vi "oax_Path Error Handle.vi"(0 "File Path (.dat)":path, 1 "Ring":u16(ring) items=["Load .wav file", "Load .dat file", "Load tachless file", "Load .ssp file"], 5 "Tacho File Path (.wav)":path, 7 "Vibration File Path (.wav)":path, 9 "Simulated File Path (.ssp)":path, 11 "error In":errorcluster) -> (4 "Error":bool, 15 "error Out":errorcluster)   [LabVIEW 2017]
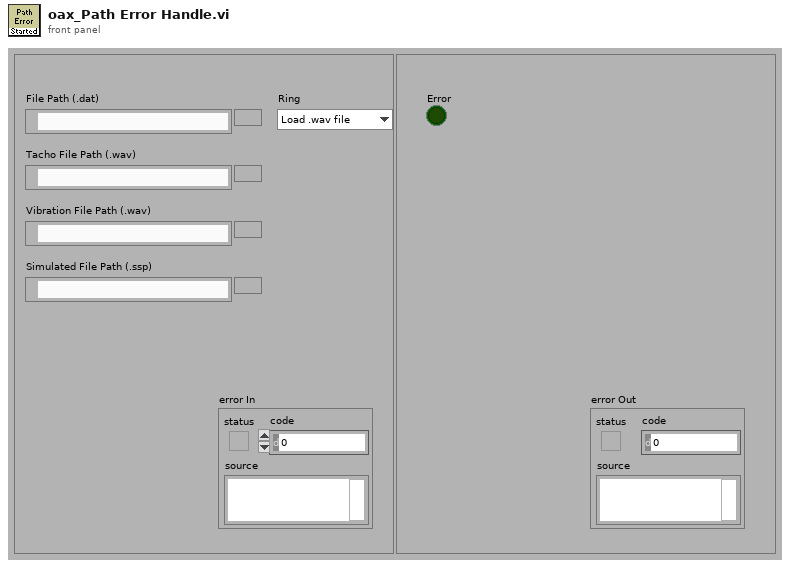
[diagram p1: front panel]
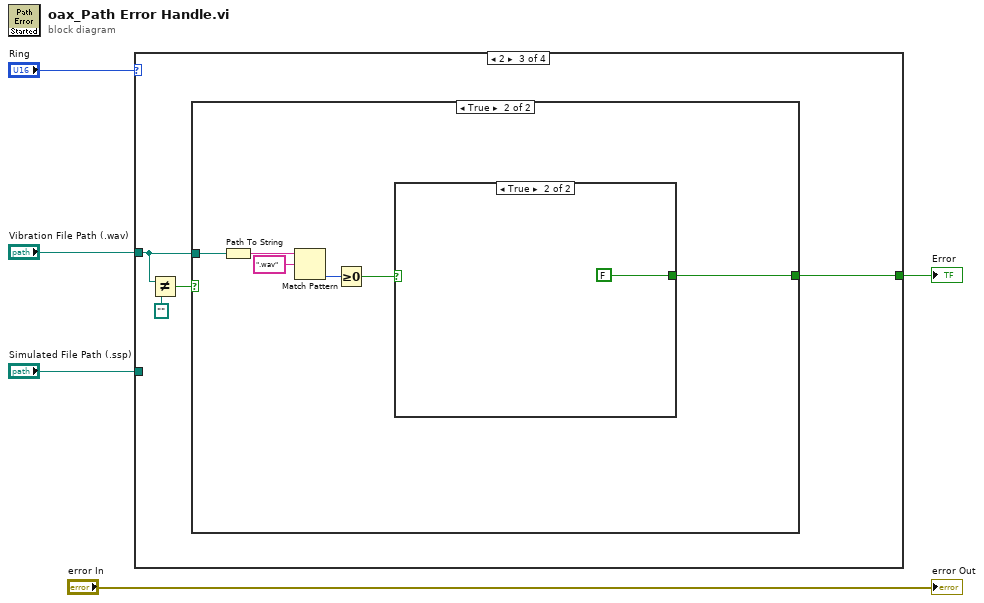
[diagram p0: block diagram]
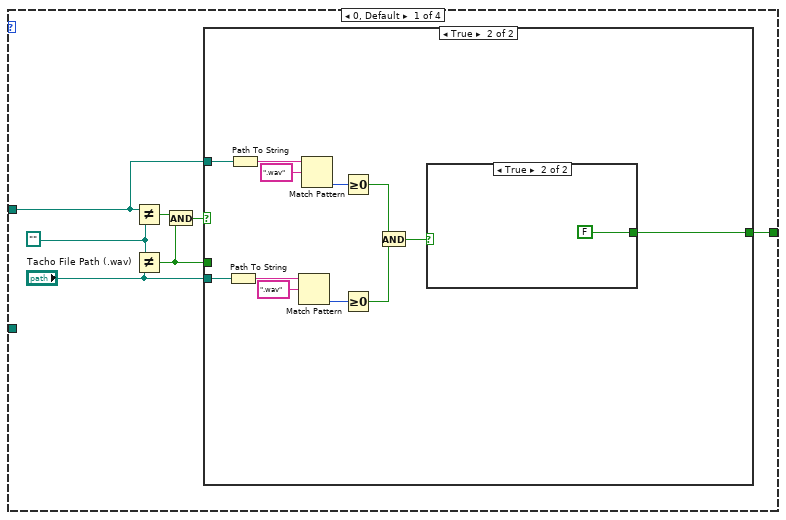
[diagram p2: hidden frame]
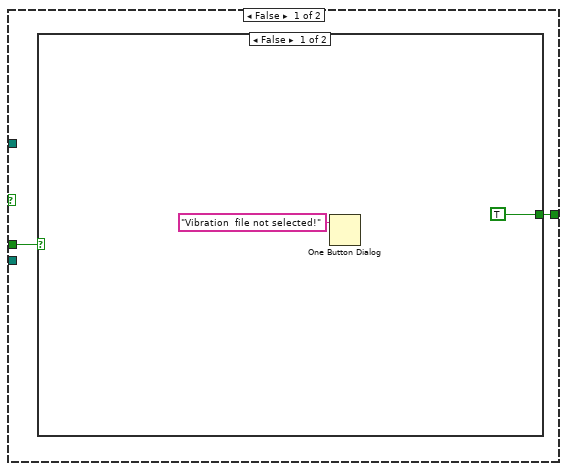
[diagram p3: hidden frame]
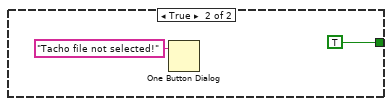
[diagram p4: hidden frame]
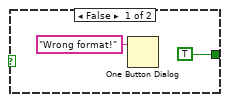
[diagram p5: hidden frame]
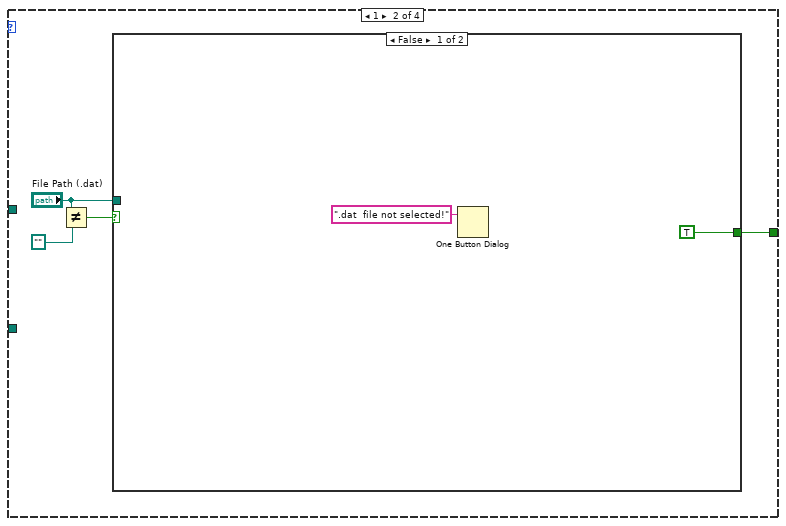
[diagram p6: hidden frame]
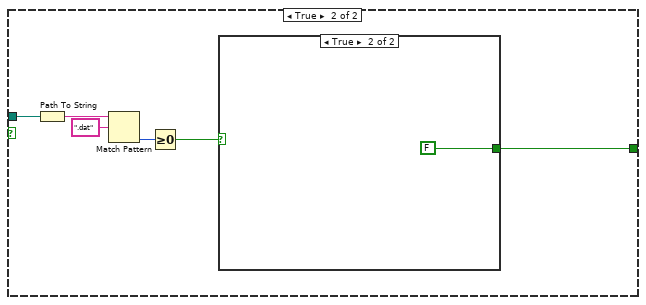
[diagram p7: hidden frame]
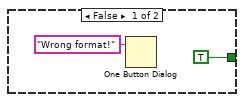
[diagram p8: hidden frame]
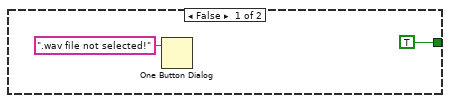
[diagram p9: hidden frame]
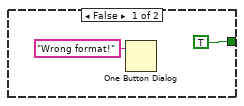
[diagram p10: hidden frame]
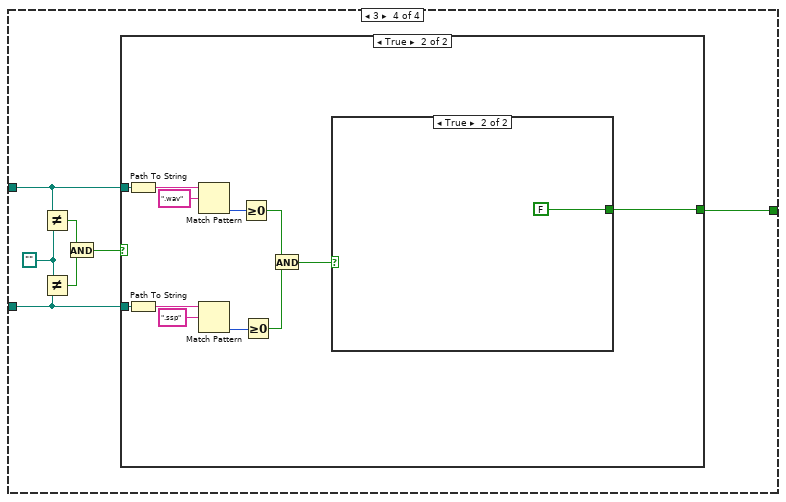
[diagram p11: hidden frame]
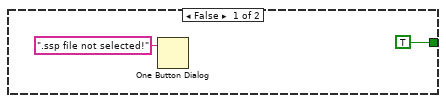
[diagram p12: hidden frame]
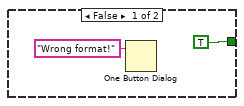
[diagram p13: hidden frame]
diagram:
  n1 = case shown="2" "Ring" {
    tunnel: [w9 w35 w49 w69] -> w4
    tunnel: "Vibration File Path (.wav)" -> [w6 _ w50 w70]
    tunnel: "Simulated File Path (.ssp)" -> [_ _ _ w64]
    frame 0, Default {
      w12 = path ""
      n2 = Not Equal?(x=w6, y=w12) -> (x != y?=w11:bool)
      n3 = Not Equal?(x=w12, y="Tacho File Path (.wav)") -> (x != y?=w8:bool)
      n4 = And(x=w11, y=w8) -> (x .and. y?=w10:bool)
      n5 = case shown="True" w10 {
        tunnel: [w13 w19] -> w9
        tunnel: w8 -> [w14 _]
        tunnel: w6 -> [_ w30]
        tunnel: "Tacho File Path (.wav)" -> [_ w29]
        frame False {
          n6 = case shown="False" w14 {
            tunnel: [TRUE ("x != y?") TRUE ("x != y?")] -> w13
            frame False {
              n7 = One Button Dialog(message="Vibration  file not selected!") -> ()  [unwired: 1 in, 1 out]
            }
            frame True {
              n8 = One Button Dialog(message="Tacho file not selected!") -> ()  [unwired: 1 in, 1 out]
            }
          }
        }
        frame True {
          n9 = Path To String(path=w29) -> (string=w25:string)
          n10 = Path To String(path=w30) -> (string=w28:string)
          n11 = Match Pattern(string=w25, regular expression=".wav") -> (offset past match=w23:i32)  [unwired: 1 in, 3 out]
          n12 = Match Pattern(string=w28, regular expression=".wav") -> (offset past match=w24:i32)  [unwired: 1 in, 3 out]
          n13 = Greater Or Equal To 0?(x=w24) -> (x >= 0?=w22:bool)
          n14 = Greater Or Equal To 0?(x=w23) -> (x >= 0?=w21:bool)
          n15 = And(x=w22, y=w21) -> (x .and. y?=w20:bool)
          n16 = case shown="True" w20 {
            tunnel: [TRUE ("x != y?") FALSE ("x != y?")] -> w19
            frame False {
              n17 = One Button Dialog(message="Wrong format!") -> ()  [unwired: 1 in, 1 out]
            }
            frame True {
            }
          }
        }
      }
    }
    frame 1 {
      n18 = Not Equal?(x="File Path (.dat)", y=path "") -> (x != y?=w36:bool)
      n19 = case shown="False" w36 {
        tunnel: [TRUE ("x != y?") w40] -> w35
        tunnel: "File Path (.dat)" -> [_ w42]
        frame False {
          n20 = One Button Dialog(message=".dat  file not selected!") -> ()  [unwired: 1 in, 1 out]
        }
        frame True {
          n21 = Path To String(path=w42) -> (string=w45:string)
          n22 = Match Pattern(string=w45, regular expression=".dat") -> (offset past match=w43:i32)  [unwired: 1 in, 3 out]
          n23 = Greater Or Equal To 0?(x=w43) -> (x >= 0?=w41:bool)
          n24 = case shown="True" w41 {
            tunnel: [TRUE ("x != y?") FALSE ("x != y?")] -> w40
            frame False {
              n25 = One Button Dialog(message="Wrong format!") -> ()  [unwired: 1 in, 1 out]
            }
            frame True {
            }
          }
        }
      }
    }
    frame 2 {
      n26 = Not Equal?(x=w50, y=path "") -> (x != y?=w51:bool)
      n27 = case shown="True" w51 {
        tunnel: w50 -> [_ w57]
        tunnel: [TRUE ("x != y?") w55] -> w49
        frame False {
          n28 = One Button Dialog(message=".wav file not selected!") -> ()  [unwired: 1 in, 1 out]
        }
        frame True {
          n29 = Path To String(path=w57) -> (string=w60:string)
          n30 = Match Pattern(string=w60, regular expression=".wav") -> (offset past match=w58:i32)  [unwired: 1 in, 3 out]
          n31 = Greater Or Equal To 0?(x=w58) -> (x >= 0?=w56:bool)
          n32 = case shown="True" w56 {
            tunnel: [TRUE ("x != y?") FALSE ("x != y?")] -> w55
            frame False {
              n33 = One Button Dialog(message="Wrong format!") -> ()  [unwired: 1 in, 1 out]
            }
            frame True {
            }
          }
        }
      }
    }
    frame 3 {
      w68 = path ""
      n34 = Not Equal?(x=w70, y=w68) -> (x != y?=w67:bool)
      n35 = Not Equal?(x=w68, y=w64) -> (x != y?=w66:bool)
      n36 = And(x=w67, y=w66) -> (x .and. y?=w65:bool)
      n37 = case shown="True" w65 {
        tunnel: w70 -> [_ w81]
        tunnel: [TRUE ("x != y?") w80] -> w69
        tunnel: w64 -> [_ w77]
        frame False {
          n38 = One Button Dialog(message=".ssp file not selected!") -> ()  [unwired: 1 in, 1 out]
        }
        frame True {
          n39 = Path To String(path=w81) -> (string=w84:string)
          n40 = Path To String(path=w77) -> (string=w78:string)
          n41 = Match Pattern(string=w84, regular expression=".wav") -> (offset past match=w82:i32)  [unwired: 1 in, 3 out]
          n42 = Match Pattern(string=w78, regular expression=".ssp") -> (offset past match=w76:i32)  [unwired: 1 in, 3 out]
          n43 = Greater Or Equal To 0?(x=w82) -> (x >= 0?=w75:bool)
          n44 = Greater Or Equal To 0?(x=w76) -> (x >= 0?=w74:bool)
          n45 = And(x=w75, y=w74) -> (x .and. y?=w73:bool)
          n46 = case shown="True" w73 {
            tunnel: [TRUE ("x != y?") FALSE ("x != y?")] -> w80
            frame False {
              n47 = One Button Dialog(message="Wrong format!") -> ()  [unwired: 1 in, 1 out]
            }
            frame True {
            }
          }
        }
      }
    }
  }
  "Error" <- w4
  "error Out" <- "error In"
